vi "Close Lockin.vi"(8 "error in (no error)":errorcluster, 11 "MeasurementSMO in":refnum<class "AFM_Litho_Plugin.IV.lvclass">) -> (0 "error out":errorcluster, 3 "MeasurementSMO out":refnum<class "AFM_Litho_Plugin.IV.lvclass">)   [LabVIEW 2019, in "AFM_Litho_Plugin.IV.lvclass"]
uses:
  AFM_Litho_Plugin.IV.lvclass
  AFM_Litho_Plugin.IV.lvclass/AFM_Litho_Plugin.IV.ctl
  <userlib>/LevyLab/Lockin-Multichannel/Instrument.Lockin/Instrument.Lockin.lvclass
  22d40c83-00b1-44b8-bf90-440ebb4134f0.vi
  22d40c83-00b1-44b8-bf90-440ebb4134f0.vi/ff40df25-0e41-4205-825d-56c19dc320b6.vi
  <vilib>/Utility/Debug Log/Display.vi
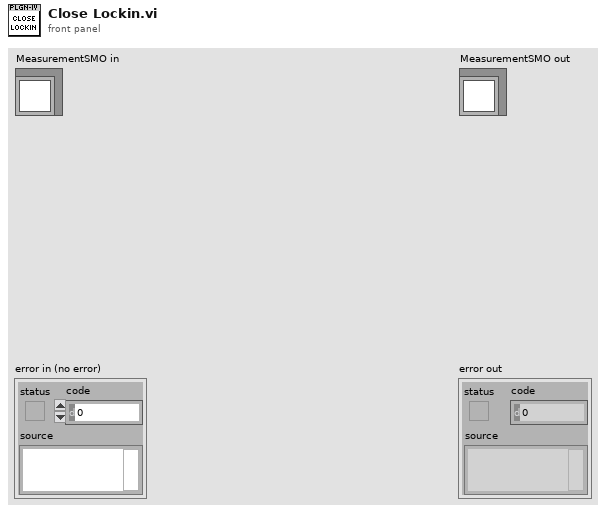
[diagram p1: front panel]
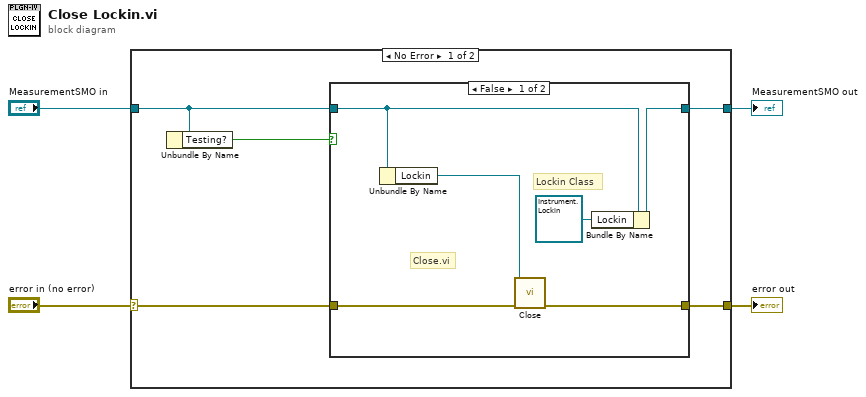
[diagram p0: block diagram]
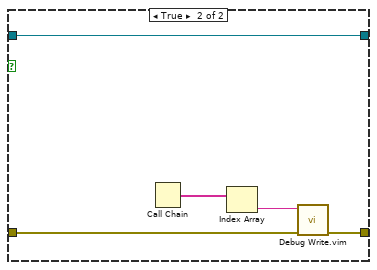
[diagram p2: hidden frame]
diagram:
  n1 = case shown="No Error" "error in (no error)" {
    selector: "error in (no error)" -> [w8 w22]
    tunnel: [w5 w22] -> w3
    tunnel: [w9 w21] -> w1
    tunnel: "MeasurementSMO in" -> [w7 w21]
    frame No Error {
      n2 = Unbundle By Name(w7) -> ("Testing?"=w6:bool)
      n3 = case shown="False" w6 {
        tunnel: [w15 w20] -> w9
        tunnel: w7 -> [w14 w20]
        tunnel: w8 -> [w11 w17]
        tunnel: [w10 w18] -> w5
        frame False {
          # "Lockin Class"
          # "Close.vi"
          n4 = Unbundle By Name(w14) -> ("Lockin"=w12:refnum<class "Instrument.Lockin.lvclass">)
          n5 = call-dynamic "Close.vi"("error in (no error)"=w11, "Instrument.Lockin in"=w12) -> ("error out"=w10:errorcluster)  [unwired: 8 in, 1 out]
          n6 = Bundle By Name(cluster=w14, "Lockin"=refnum<class "Instrument.Lockin.lvclass"> refnum) -> (w15:refnum<class "AFM_Litho_Plugin.IV.lvclass">)
        }
        frame True {
          n7 = Call Chain() -> (call chain=w19:string[])
          n8 = Index Array(array=w19) -> (element=w16:string)  [unwired: 1 in]
          n9 = call "Debug Write.vim"("error in (no error)"=w17, "value"=w16) -> ("error out"=w18:errorcluster)  [unwired: 9 in]
        }
      }
    }
    frame Error {
    }
  }
  "error out" <- w3
  "MeasurementSMO out" <- w1
